vi "Read Enabled Channels.vi"(8 "error in (no error)":errorcluster, 11 "No-op Parser in":refnum<class "No-op Parser.lvclass">) -> (0 "error out":errorcluster, 2 "Enabled Channels":string[](array[string]), 3 "No-op Parser out":refnum<class "No-op Parser.lvclass">)   [LabVIEW 2015, in "No-op Parser.lvclass"]
doc: "No-op Parser.lvclass:Read Enabled Channels.vi\n\nThis VI returns the list of channel names that are enabled for the No-op Parser class..\n\nInstrument Communication Module Version 1.0\nJanuary, 2018 Original Code Consulting David Thomson\n www.originalcode.com"
uses:
  No-op Parser.lvclass
  No-op Parser.lvclass/No-op Parser.ctl
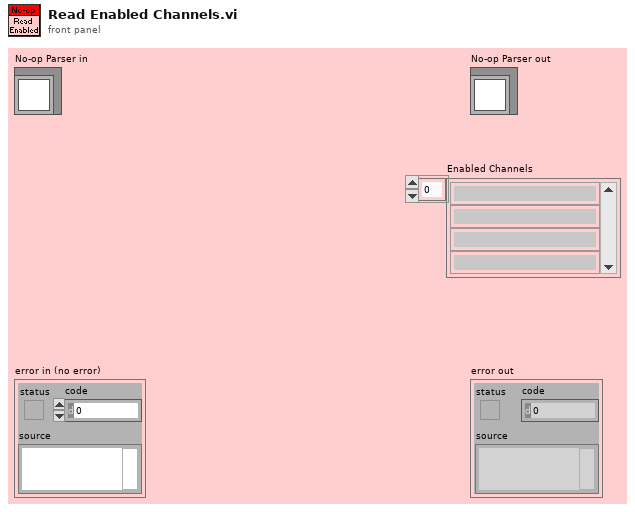
[diagram p1: front panel]
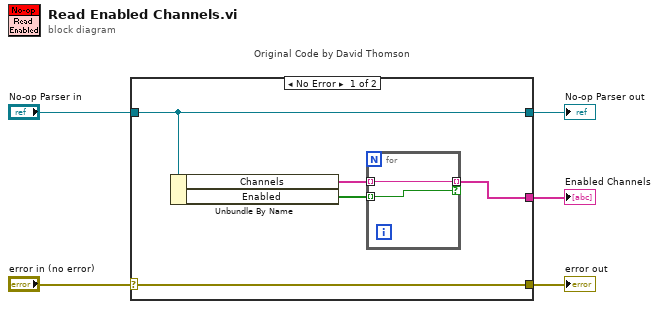
[diagram p0: block diagram]
diagram:
  n1 = case "Original Code by David Thomson" shown="No Error" "error in (no error)" {
    selector: "error in (no error)" -> [w10 w13]
    tunnel: [w10 w13] -> w4
    tunnel: [w9 w14] -> w2
    tunnel: "No-op Parser in" -> [w9 w14]
    tunnel: [w6 _] -> w1
    frame No Error {
      n2 = Unbundle By Name(w9) -> ("Channels"=w8:string[], "Enabled"=w7:bool[])
      n3 = for {
        tunnel: [w12] -> w6 mode=indexing if=w11
        tunnel: w8 -> [w12] mode=indexing
        tunnel: w7 -> [w11] mode=indexing
      }
    }
    frame Error {
    }
  }
  "error out" <- w4
  "No-op Parser out" <- w2
  "Enabled Channels" <- w1
